vi "CheckReadParamValIsEmpty.vi"(9 "Parameter":string, 11 "Input Value":string) -> (2 "concatenated string":string)   [LabVIEW 2017, in "PlayNitrideCameraComponet1010_4.lvlib"]
uses:
  <userlib>/PlayNitrideCameraComponet1010_4/PlayNitrideCameraComponet1010_4.lvlib
panel:
  in  "Reference String":string
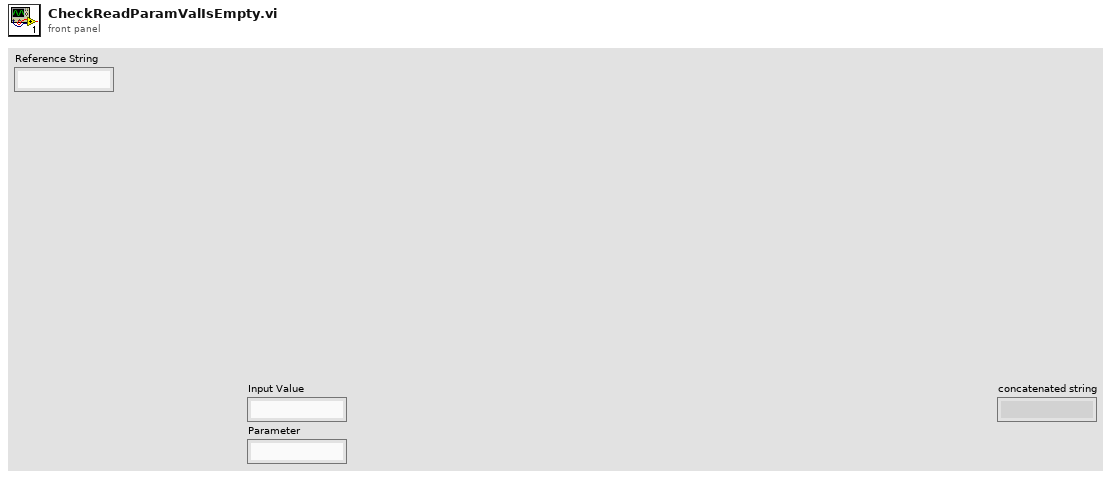
[diagram p1: front panel]
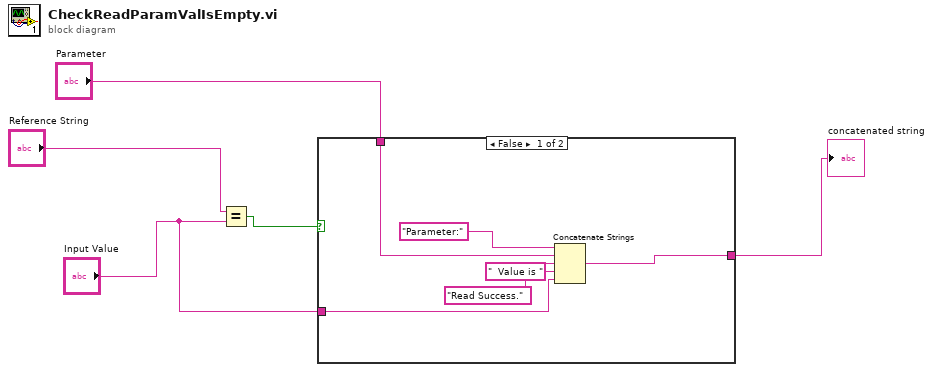
[diagram p0: block diagram]
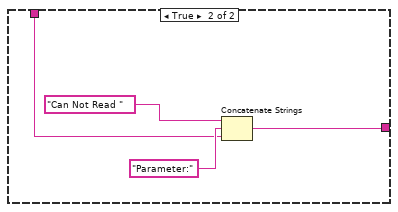
[diagram p2: hidden frame]
diagram:
  n1 = Equal?(x="Reference String", y="Input Value") -> (x = y?=w5:bool)
  n2 = case shown="False" w5 {
    tunnel: "Parameter" -> [w9 w12]
    tunnel: [w8 w14] -> w3
    tunnel: "Input Value" -> [w6 _]
    frame False {
      n3 = Concatenate Strings("Parameter:" ("Error Output.source"), w9, "Read Success." ("string"), "  Value is " ("string"), w6) -> (w8:string)
    }
    frame True {
      n4 = Concatenate Strings("Can Not Read " ("Error Output.source"), "Parameter:" ("string"), w12) -> (w14:string)
    }
  }
  "concatenated string" <- w3
